vi "streak calculate lengths.vi"(9 "max index":i32, 10 "streak step (fraction)":dbl, 11 "streak length (fraction)":dbl) -> (2 "streak step (points)":i32, 3 "streak length (points)":i32)   [LabVIEW 2020]
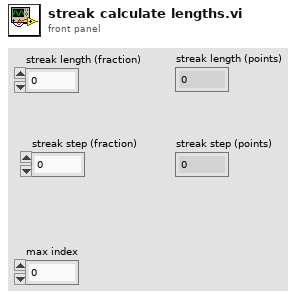
[diagram p1: front panel]
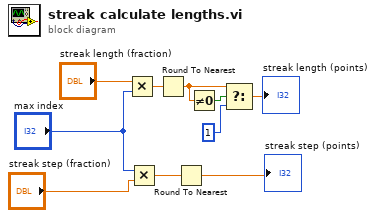
[diagram p0: block diagram]
diagram:
  n1 = Multiply(x="streak length (fraction)", y="max index") -> (x*y=w4:dbl)
  n2 = Multiply(x="max index", y="streak step (fraction)") -> (x*y=w5:dbl)
  n3 = Round To Nearest(number=w4) -> (nearest integer value=w7:dbl)
  n4 = Round To Nearest(number=w5) -> (nearest integer value=→"streak step (points)":dbl)
  n5 = Not Equal To 0?(x=w7) -> (x != 0?=w6:bool)
  n6 = Select(t=w7, s=w6, f=1) -> (s? t:f=→"streak length (points)":dbl)
